vi "Configure Trigger.vi"   [LabVIEW 2010, in "Agilent DSO1000 Series.lvlib"]
doc: "Selects the type of trigger."
uses:
  <instrlib>/Agilent DSO1000 Series/Agilent DSO1000 Series.lvlib
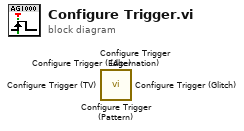
[diagram p0: block diagram]
diagram:
  n1 = call <instrlib>:"Configure Trigger (Pattern).vi"() -> ()  [unwired: 14 in, 2 out]
  n2 = call <instrlib>:"Configure Trigger (Alternation).vi"() -> ()  [unwired: 14 in, 2 out]
  n3 = call <instrlib>:"Configure Trigger (TV).vi"() -> ()  [unwired: 14 in, 2 out]
  n4 = call <instrlib>:"Configure Trigger (Glitch).vi"() -> ()  [unwired: 14 in, 2 out]
  n5 = call <instrlib>:"Configure Trigger (Edge).vi"() -> ()  [unwired: 14 in, 2 out]
